vi "pathtracking.vi"(8 "x":dbl, 11 "y":dbl) -> (3 "R":dbl)   [LabVIEW 2012]
uses:
  G_NAV.vi
  G_VEH.vi
  G_PATH.vi
  <vilib>/Analysis/NI_AALBase.lvlib
  <vilib>/Analysis/baseanly.llb/Real Determinant.vi
  <vilib>/Analysis/baseanly.llb/Real Inverse Matrix.vi
  <vilib>/Analysis/baseanly.llb/A x Vector.vi
panel:
  out "Waveform Graph":dbl[](graph)
  out "Array 2":dbl[](array[numeric])
  out "Array":dbl[](array[numeric])
  out "x*y 2":dbl[](array[numeric])
  out "sqrt(x)":dbl[](array[numeric])
  out "x*y":dbl[](array[numeric])
  out "map_track 2":dbl[][](array[numeric])
  out "sum":dbl
  out "M6006":T1={"GPSTime"=22892800.0, "attitude[2]"=-0.6123908, "lcc[0]"=-970.47205, "lcc[1]"=200.52362, "heading_GPS"=-0.6106907} {"GPSTime" format="%#_6f"}
  out "stack":bool=TRUE
  out "lw":dbl=0.4
  out "tic":u32=313769281
  out "reverse":bool
  out "map_track":dbl[][](array[numeric])=[[-0.6687401515638595, -3.551350516814976], [-1.1601880006125764, -3.4580278333550782], [-1.6512488590649952, -3.3629580799680854], [-2.1418835557610314, -3.265964418362822], [-2.6320529195405924, -3.1668700102479344], [-3.12171777924361, -3.0654980173321356], [-3.6108389637099756, -2.961671601324125], [-4.250355012057505, -2.8217269001890974], [-4.733554194697693, -2.693195492254268]]
  out "track":dbl[][](array[numeric])=[[-0.6687401515638595, -3.551350516814976], [-1.1601880006125764, -3.4580278333550782], [-1.6512488590649952, -3.3629580799680854], [-2.1418835557610314, -3.265964418362822], [-2.6320529195405924, -3.1668700102479344], [-3.12171777924361, -3.0654980173321356], [-3.6108389637099756, -2.961671601324125], [-4.250355012057505, -2.8217269001890974], [-4.733554194697693, -2.693195492254268], [-5.215089885143842, -2.558342659026822], [-5.693483406062963, -2.4115492889016945], [-6.167256080122039, -2.24719627027381], [-6.634929229988109, -2.059664491538052], [-7.095024178328142, -1.8433348410893422], [-7.546062247809149, -1.5925882073226139], [-7.98656476109811, -1.301805478632852], [-8.415053040862054, -0.9653675434148765], [-8.830048409767974, -0.5776552900636165], [-9.230072190482858, -0.133049606974057], [-9.61364570567371, 0.3740686174589265], [-9.97929027800753, 0.949318494840405], [-10.386059580111024, 1.7242186788508236], [-10.53357405922493, 2.2019628347040774], [-10.66851200140239, 2.6835902739278463], [-10.772007434080049, 3.1749262819640283], [-10.825194384694537, 3.6817961442544633], [-10.809206880682517, 4.210025146240928], [-10.705178949480636, 4.765438573365376], [-10.494244618525542, 5.353861711069529], [-10.157537915253862, 5.981119844795286], [-9.676192867102248, 6.653038259984428], [-8.946295802610212, 7.461572105302583], [-8.539313408094966, 7.752602995705581], [-8.110420661696207, 8.015244834208291], [-7.660232732059987, 8.25029468946181], [-7.189364787832295, 8.458549630117131], [-6.698431997659123, 8.640806724825243], [-6.188049530186491, 8.797863042237132], [-5.658832554060375, 8.930515651003796], [-5.11139623792681, 9.039561619776274], [-4.546355750431802, 9.12579801720561], [-3.9643262602213256, 9.190021911942688], [-3.3659229359414162, 9.233030372638604], [-2.7517609462380523, 9.25562046794435], [-2.122455459757251, 9.258589266510917], [-1.4786216451450183, 9.242733836989292], [-0.8208746710473604, 9.208851248030518], [-0.1498297061102689, 9.157738568285591], [0.5338980810202378, 9.090192866405497], [1.229693521698167, 9.007011211041284], [1.9369414472775146, 8.908990670843883], [2.6550266891122614, 8.796928314464337], [3.383334078556428, 8.671621210553642], [4.121248446963983, 8.53386642776284], [4.868154625688948, 8.384461034742866], [5.623437446085289, 8.224202100144819], [6.386481739507029, 8.053886692619635], [7.156672337308164, 7.874311880818305], [7.838146127104554, 7.70968069378327], [8.321781606815595, 7.582803343212244], [8.805290536895978, 7.45544776805299], [9.287663918083021, 7.323801011645703], [9.76789275111402, 7.18405011733063], [10.244968036726283, 7.032382128447967], [10.717880775657084, 6.864984088337955], [11.18562196864372, 6.678043040340844], [11.647182616423507, 6.4677460277968315], [12.101553719733744, 6.230280094046104], [12.547726279311707, 5.961832282428966], [12.984691295894704, 5.658589636285609], [13.411439770220039, 5.3167391989562285], [13.939637565704926, 4.818324597988705], [14.177469695018669, 4.377621822306417], [14.370305638929839, 3.9092831916317614], [14.522185803389362, 3.415790251277338], [14.637150594348116, 2.8996245465557346], [14.719240417757044, 2.363267622779441], [14.77249567956704, 1.8092010252611073], [14.800956785728996, 1.2399062993133256], [14.808664142193827, 0.6578649902486369], [14.799658154912459, 0.06555864337958095], [14.777979229835777, -0.5345311959811911]]
  out "xyhc":T2={"c_idx"=71, "xc"=-91.48037348905598, "yc"=-434.27857700428615, "hc"=-0.4484199308552679, "xc_path"=12.43286899562552}
  in  "margin":dbl
  out "vr":dbl=0.75
  out "vf":dbl=3.5
  out "vw":dbl=0.9025
  out "ymax":dbl=12.0
  out "ymin":dbl=-6.0
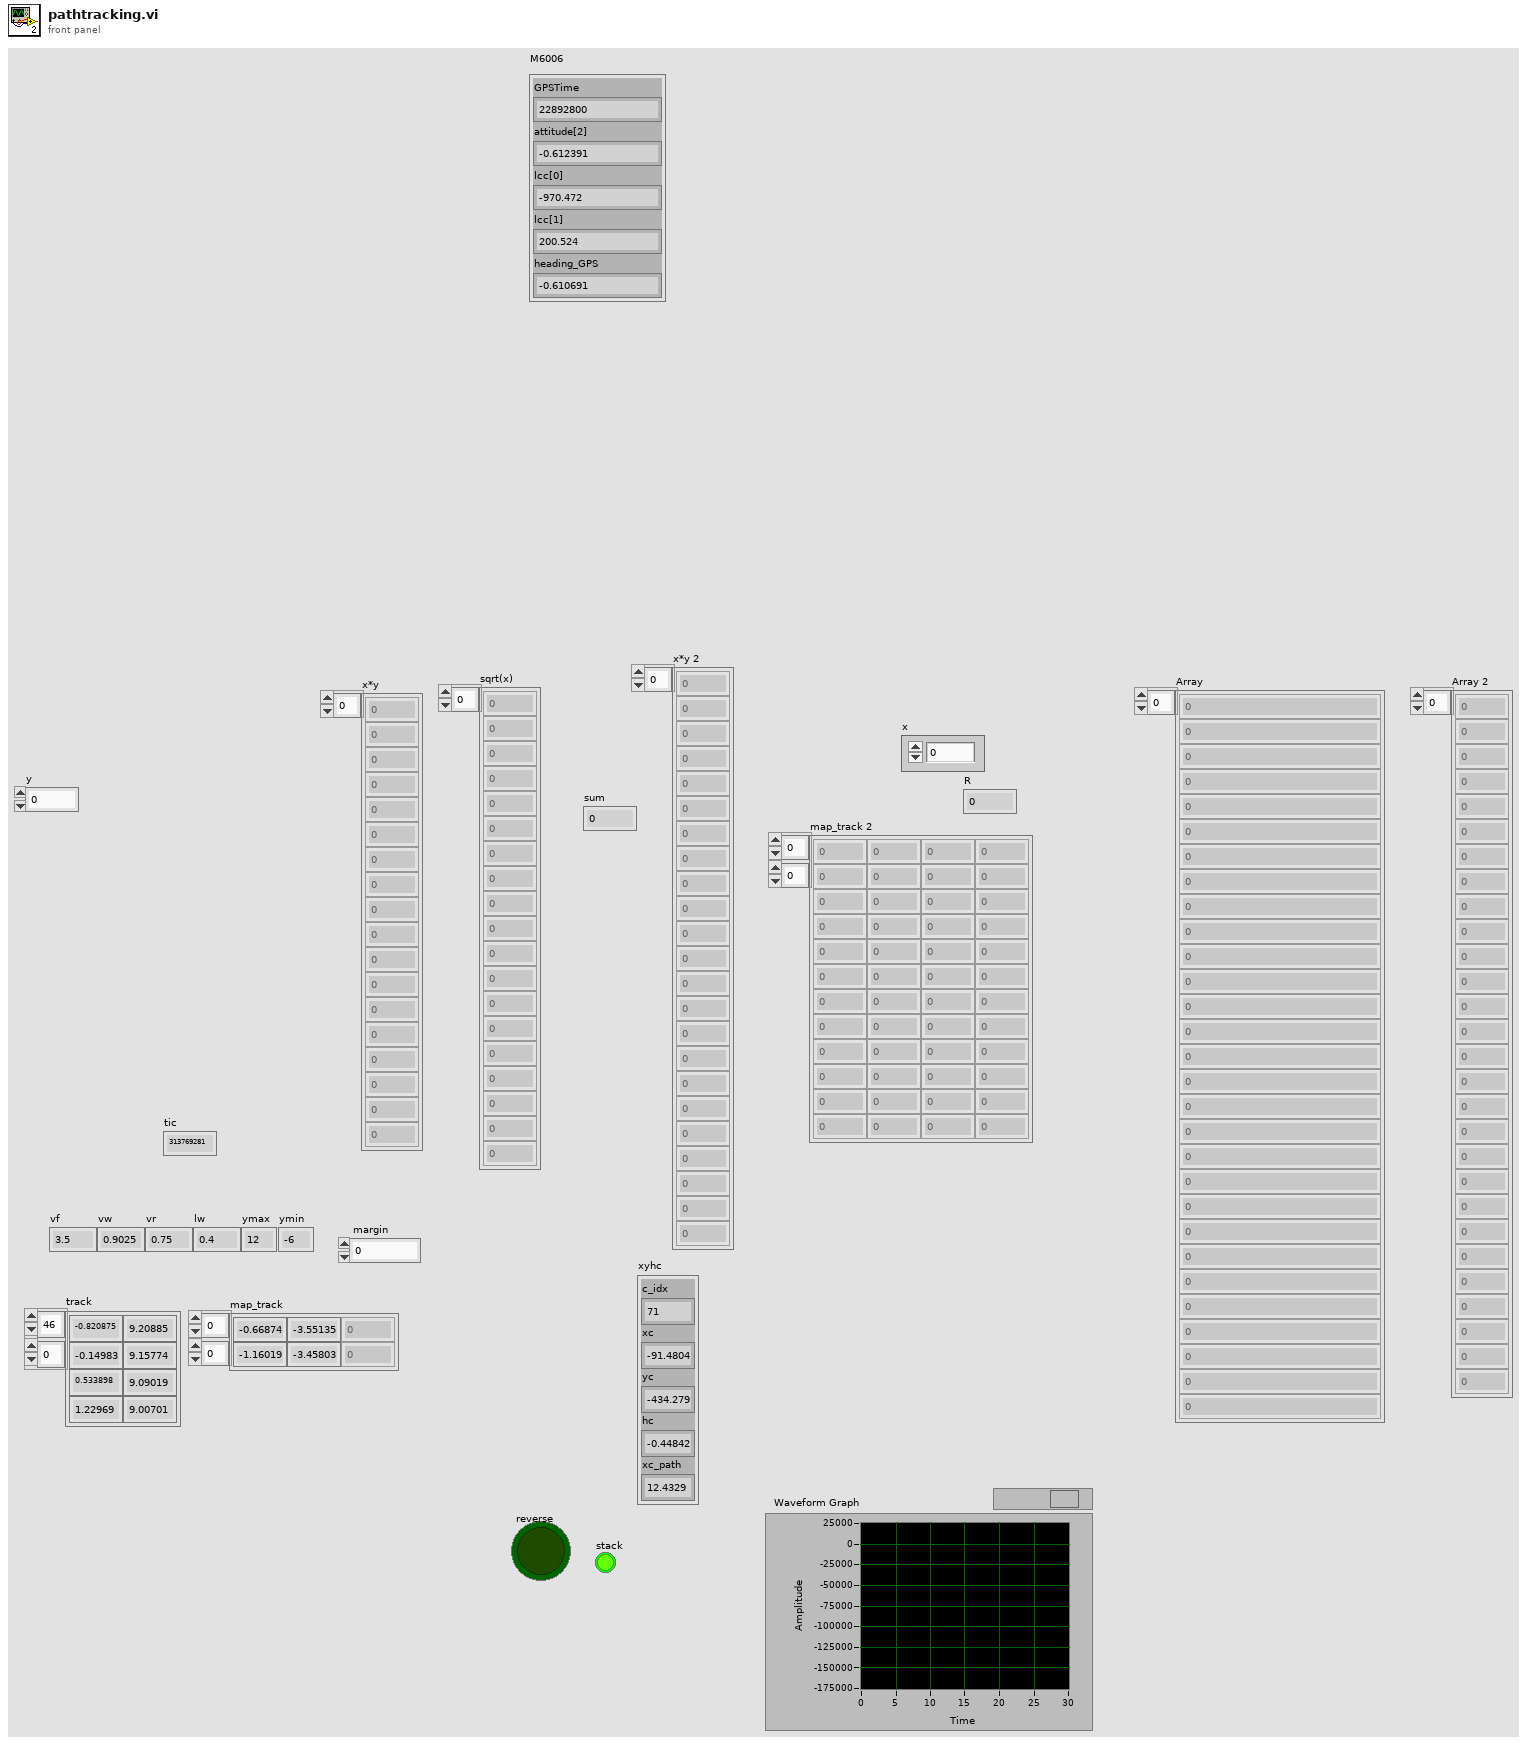
[diagram p1: front panel]
types:
  T1 = cluster{"GPSTime":dbl, "attitude[2]":sgl, "lcc[0]":sgl, "lcc[1]":sgl, "heading_GPS":sgl}
  T2 = cluster{"c_idx":i32, "xc":dbl, "yc":dbl, "hc":dbl, "xc_path":dbl}
  T3 = enum32{"General", "Positive Definite", "Lower Triangular", "Upper Triangular"}
  T4 = cluster{"GPSTime":dbl, "attitude[2]":dbl, "lcc[0]":dbl, "lcc[1]":dbl, "heading_GPS":dbl}
  T5 = cluster{"Steer_input":dbl, "Steer_output":dbl, "VS_des":dbl, "VS_can":dbl, "heading":dbl, "auto":bool, "run":bool, "x":dbl, "y":dbl}
  T6 = cluster{"idx":i32, "x":dbl, "y":dbl, "h":dbl, "x_path":dbl}
  T7 = typedef "NI_Matrix.lvlib/RealMatrix.ctl" = dbl[][]
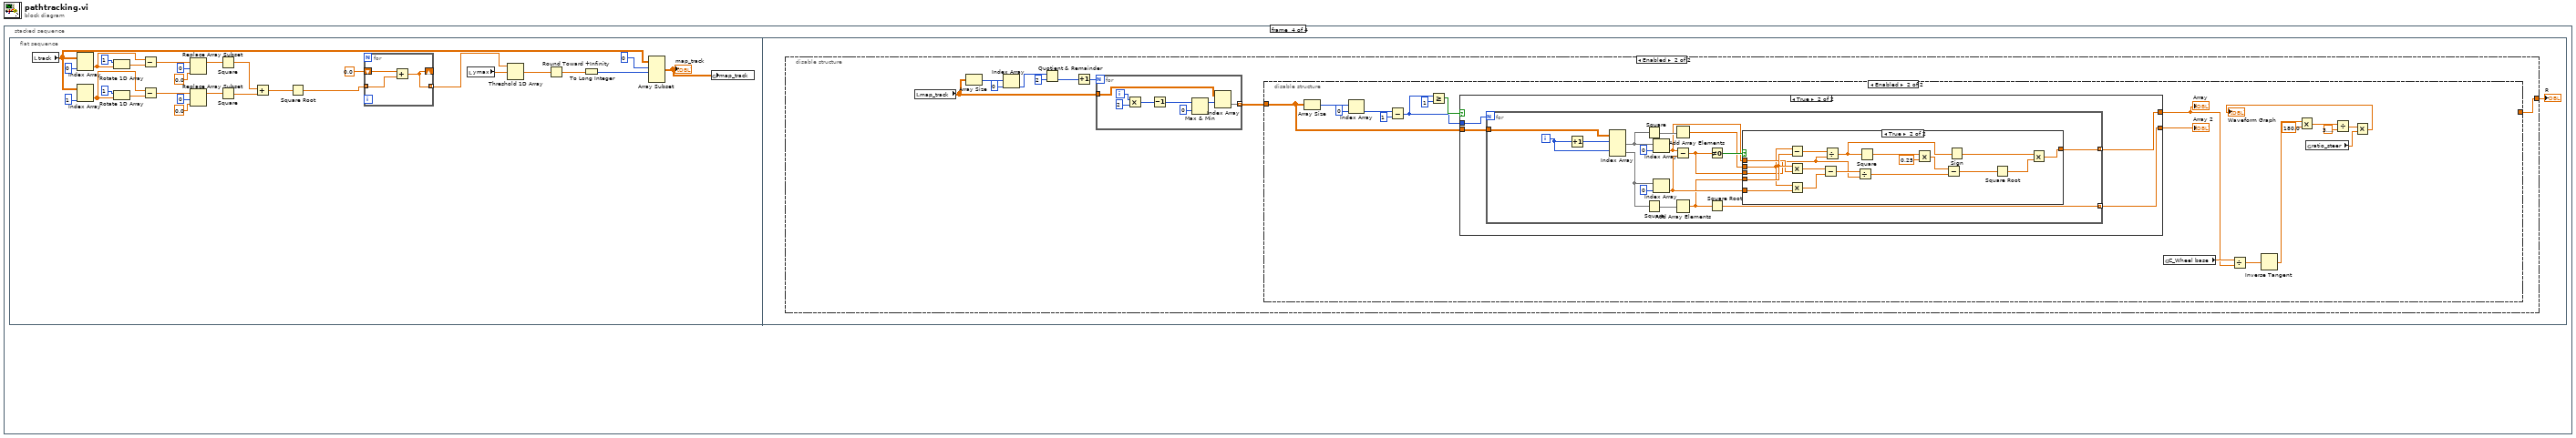
[diagram p0: block diagram]
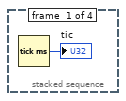
[diagram p2: hidden frame]
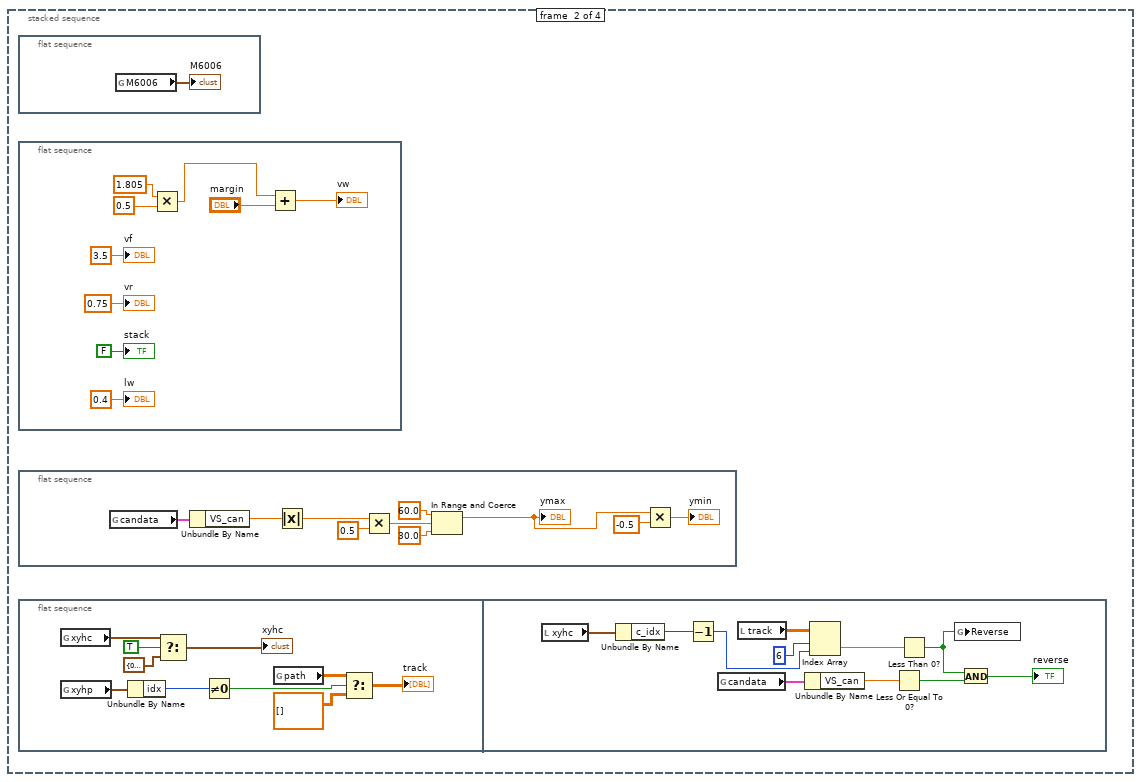
[diagram p3: hidden frame]
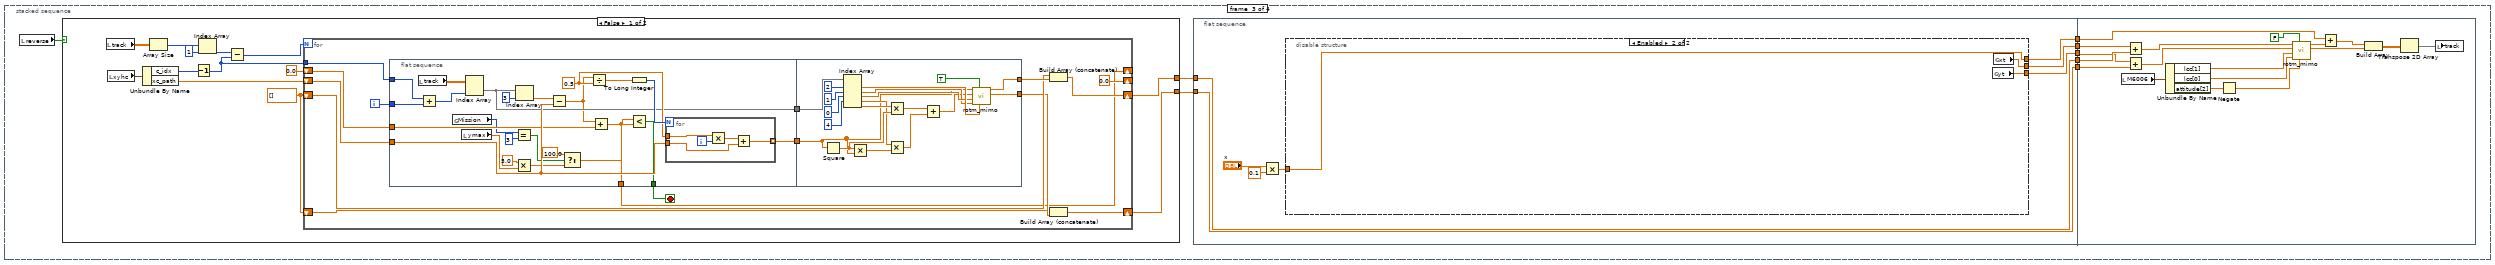
[diagram p4: hidden frame]
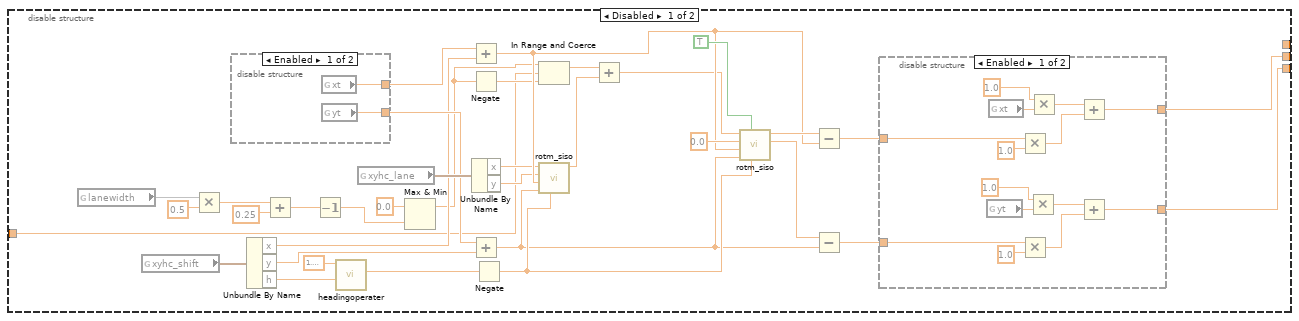
[diagram p5: hidden frame]
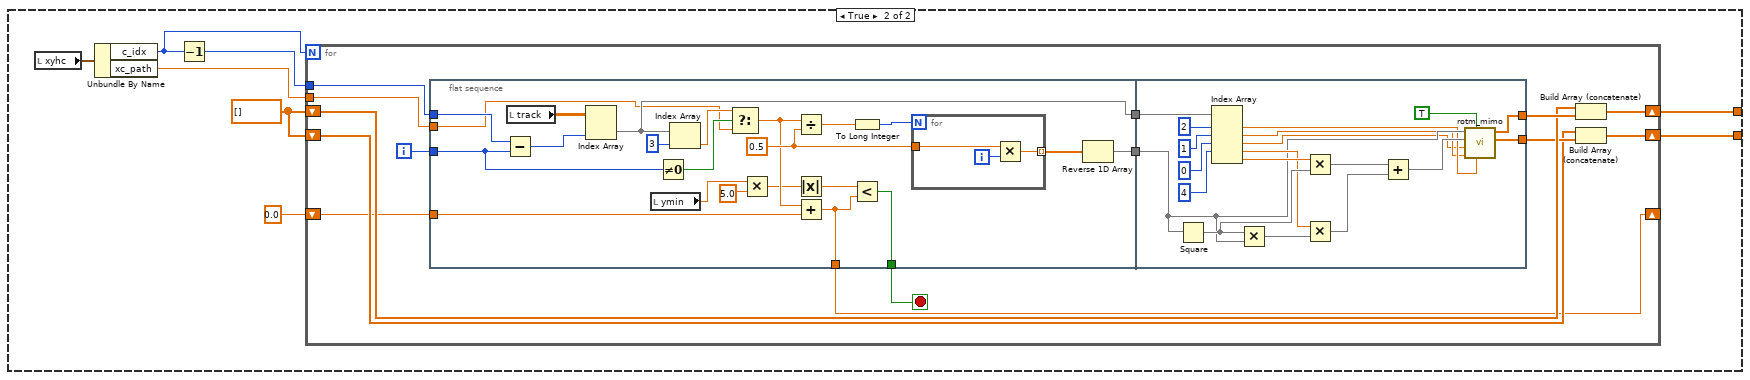
[diagram p8: hidden frame]
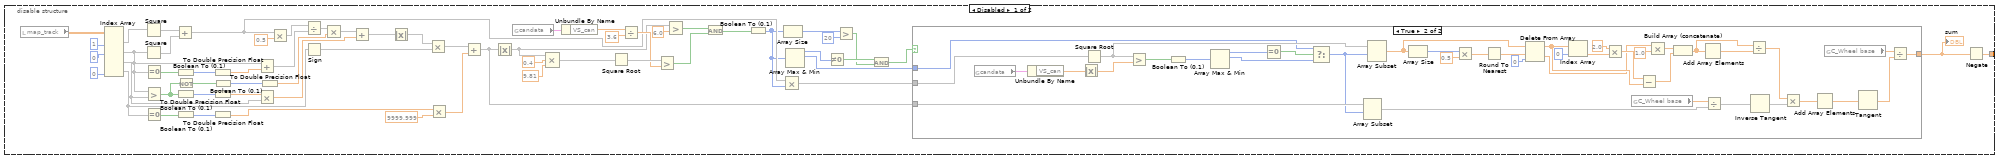
[diagram p9: hidden frame]
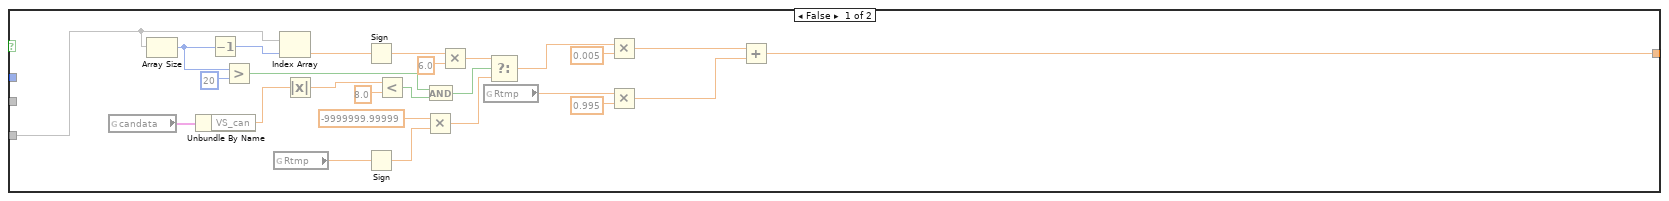
[diagram p10: hidden frame]
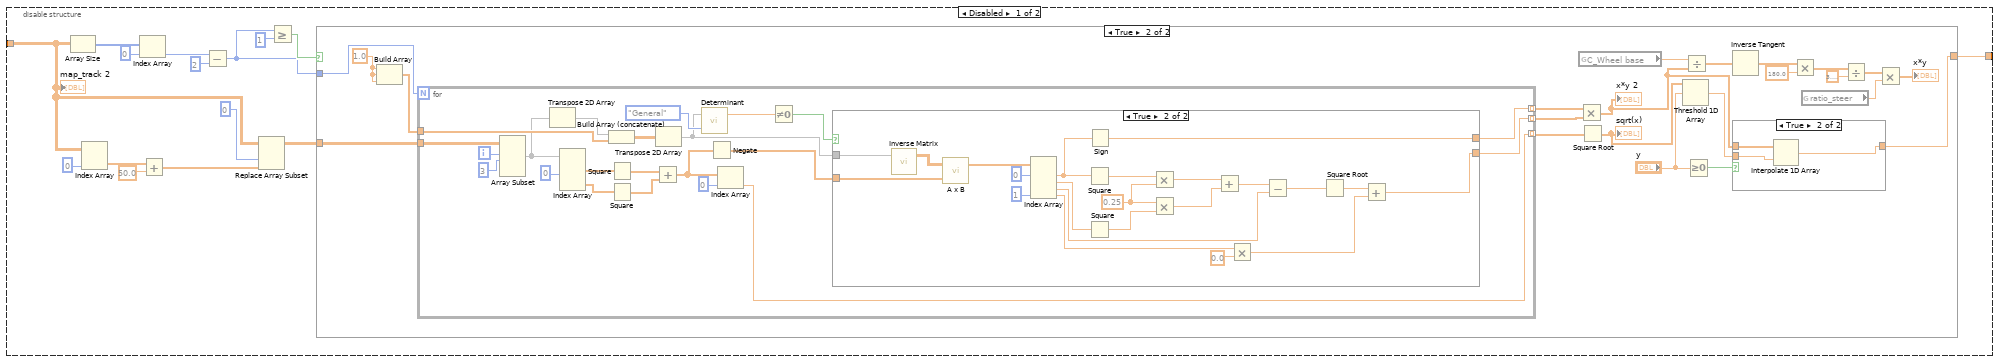
[diagram p11: hidden frame]
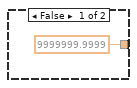
[diagram p12: hidden frame]
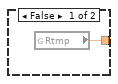
[diagram p13: hidden frame]
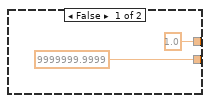
[diagram p14: hidden frame]
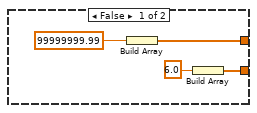
[diagram p15: hidden frame]
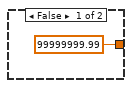
[diagram p16: hidden frame]
diagram:
  n1 = stacked-sequence {
    frame #0 {
      n2 = Tick Count (ms)() -> (millisecond timer value=→"tic":u32)
    }
    frame #1 {
      n3 = flat-sequence {
        frame #0 {
          n4 = global read "G_NAV.vi" "M6006"() -> (→"M6006":T4)
        }
      }
      n5 = flat-sequence {
        frame #0 {
          n6 = Multiply(x=1.805 ("width"), y=0.5) -> (x*y=w24:dbl)
          n7 = Add(x=w24, y="margin") -> (x+y=→"vw":dbl)
          "lw" <- 0.4 ("width")
          "vf" <- 3.5 ("af")
          "vr" <- 0.75 ("ar")
          "stack" <- FALSE
        }
      }
      n8 = flat-sequence {
        frame #0 {
          n9 = global read "G_VEH.vi" "candata"() -> (w41:T5)
          n10 = Unbundle By Name(w41) -> ("VS_can"=w38:dbl)
          n11 = Absolute Value(x=w38) -> (abs(x)=w34:dbl)
          n12 = Multiply(x=w34, y=0.5 ("vgain")) -> (x*y=w33:dbl)
          n13 = In Range and Coerce(upper limit=60.0, x=w33, lower limit=30.0 ("y")) -> (coerced(x)=w37:dbl)  [unwired: 1 out]
          "ymax" <- w37
          n14 = Multiply(x=w37, y=-0.5) -> (x*y=→"ymin":dbl)
        }
      }
      n15 = flat-sequence {
        frame #0 {
          n16 = global read "G_VEH.vi" "xyhc"() -> (w9:T6)
          n17 = global read "G_VEH.vi" "xyhp"() -> (w4:T6)
          n18 = Unbundle By Name(w4) -> ("idx"=w3:i32)
          n19 = Select(t=w9, s=TRUE ("B_track"), f=T2 {"c_idx"=0, "xc"=0.0, "yc"=0.0, "hc"=0.0, "xc_path"=0.0}) -> (s? t:f=→"xyhc":T2)
          n20 = Not Equal To 0?(x=w3) -> (x != 0?=w2:bool)
          n21 = global read "G_PATH.vi" "path"() -> (w5:dbl[][])
          n22 = Select(t=w5, s=w2, f=dbl[][] []) -> (s? t:f=→"track":dbl[][])
        }
        frame #1 {
          n23 = local read "xyhc"() -> (w21:T2)
          n24 = Unbundle By Name(w21) -> ("c_idx"=w19:i32)
          n25 = Decrement(x=w19) -> (x-1=w20:i32)
          n26 = global read "G_VEH.vi" "candata"() -> (w15:T5)
          n27 = local read "track"() -> (w22:dbl[][])
          n28 = Unbundle By Name(w15) -> ("VS_can"=w16:dbl)
          n29 = Index Array(array=w22, index (row)=6, index (col)=w20) -> (element=w17:dbl)
          n30 = Less Or Equal To 0?(x=w16) -> (x <= 0?=w13:bool)
          n31 = Less Than 0?(x=w17) -> (x < 0?=w14:bool)
          n32 = global write "G_VEH.vi" "Reverse"(w14) -> ()
          n33 = And(x=w14, y=w13) -> (x .and. y?=→"reverse":bool)
        }
      }
    }
    frame #2 {
      n34 = local read "reverse"() -> (w48:bool)
      n35 = case shown="False" w48 {
        tunnel: [w136 w211] -> w50
        tunnel: [w135 w210] -> w49
        frame False {
          w138 = dbl[] [] ("x")
          n36 = local read "track"() -> (w133:dbl[][])
          n37 = local read "xyhc"() -> (w132:T2)
          n38 = Unbundle By Name(w132) -> ("c_idx"=w143:i32, "xc_path"=w131:dbl)
          n39 = Array Size(array=w133) -> (size(s)=w142:i32[])
          n40 = Decrement(x=w143) -> (x-1=w139:i32)
          n41 = Index Array(array=w142, index=1) -> (element=w140:i32)
          n42 = Subtract(x=w140, y=w139) -> (x-y=w137:i32)
          n43 = for {
            N: w137 -> [_]
            tunnel: w139 -> [w157]
            shift-right: [0.0 ("xc_path")] -> _
            shift-left: w131 -> [w155]
            shift-right: [w150] -> w136
            shift-left: w138 -> [w151]
            shift-right: [w147] -> w135
            shift-left: w138 -> [w148]
            shift-right: [w145] -> _
            shift-left: 0.0 -> [w146]
            i -> [w158]
            stop <- w144 stop-if-true
            n44 = flat-sequence {
              tunnel: w158 -> [w182]
              tunnel: w157 -> [w181]
              tunnel: w155 -> [w175]
              tunnel: [w173] -> w154
              tunnel: [w172] -> w153
              tunnel: w146 -> [w170]
              tunnel: [w169] -> w145
              tunnel: [w168] -> w144
              tunnel: w154 -> [w188]
              tunnel: w153 -> [w199]
              tunnel: [w195] -> w152
              tunnel: [w194] -> w149
              frame #0 {
                w174 = 0.5 ("y")
                n45 = local read "track"() -> (w167:dbl[][])
                n46 = Add(x=w181, y=w182) -> (x+y=w180:i32)
                n47 = global read "G_PATH.vi" "Mission"() -> (w159:i32)
                n48 = local read "ymax"() -> (w166:dbl)
                n49 = Index Array(array=w167, index (col)=w180) -> (element=w172:dbl[])  [unwired: 1 in]
                n50 = Equal?(x=w159, y=3) -> (x = y?=w164:bool)
                n51 = Multiply(x=5.0 ("f"), y=w166) -> (x*y=w161:dbl)
                n52 = Index Array(array=w172, index=3) -> (element=w178:dbl)
                n53 = Subtract(x=w178, y=w175) -> (x-y=w171:dbl)
                n54 = Select(t=100.0 ("x"), s=w164, f=w161) -> (s? t:f=w160:dbl)
                n55 = Divide(x=w171, y=w174) -> (x/y=w177:dbl)
                n56 = Add(x=w171, y=w170) -> (x+y=w169:dbl)
                n57 = To Long Integer(number=w177) -> (32bit integer=w176:i32)
                n58 = Less?(x=w160, y=w169) -> (x < y?=w168:bool)
                n59 = for {
                  N: w176 -> [_]
                  tunnel: w175 -> [w183]
                  tunnel: w174 -> [w186]
                  tunnel: [w185] -> w173 mode=indexing
                  i -> [w187]
                  n60 = Multiply(x=w186, y=w187) -> (x*y=w184:dbl)
                  n61 = Add(x=w184, y=w183) -> (x+y=w185:dbl)
                }
              }
              frame #1 {
                n62 = Square(x=w188) -> (x^2=w204:dbl[])
                n63 = Index Array(array=w199, index #1=2 ("index"), index #2=1 ("index"), index #3=0 ("index"), index #4=4 ("index")) -> (element #1=w192:dbl, element #2=w190:dbl, element #3=w191:dbl, element #4=w203:dbl, element #5=w205:dbl)  [unwired: 1 in]
                n64 = Multiply(x=w204, y=w188) -> (x*y=w202:dbl[])
                n65 = Multiply(x=w205, y=w204) -> (x*y=w201:dbl[])
                n66 = Multiply(x=w203, y=w202) -> (x*y=w200:dbl[])
                n67 = Add(x=w201, y=w200) -> (x+y=w189:dbl[])
                n68 = call "rotm_mimo.vi"("angle[rad]"=w192, "reverse"=TRUE, "y0"=w190, "x0"=w191, "y"=w189, "x"=w188) -> ("Y"=w194:dbl[], "X"=w195:dbl[])  [unwired: 2 in, 2 out]
              }
            }
            n69 = Build Array (concatenate)(w151, w152) -> (w150:dbl[])
            n70 = Build Array (concatenate)(w148, w149) -> (w147:dbl[])
          }
        }
        frame True {
          w212 = dbl[] [] ("x")
          n71 = local read "xyhc"() -> (w207:T2)
          n72 = Unbundle By Name(w207) -> ("c_idx"=w209:i32, "xc_path"=w213:dbl)
          n73 = Decrement(x=w209) -> (x-1=w214:i32)
          n74 = for {
            N: w209 -> [_]
            tunnel: w214 -> [w227]
            shift-right: [w221] -> w211
            shift-left: w212 -> [w222]
            shift-right: [w218] -> w210
            shift-left: w212 -> [w219]
            tunnel: w213 -> [w226]
            shift-right: [w216] -> _
            shift-left: 0.0 -> [w217]
            i -> [w228]
            stop <- w215 stop-if-true
            n75 = flat-sequence {
              tunnel: w228 -> [w243]
              tunnel: w227 -> [w250]
              tunnel: w226 -> [w240]
              tunnel: [w238] -> w225
              tunnel: [w244] -> w224
              tunnel: w217 -> [w236]
              tunnel: [w235] -> w216
              tunnel: [w234] -> w215
              tunnel: w225 -> [w258]
              tunnel: w224 -> [w265]
              tunnel: [w261] -> w223
              tunnel: [w260] -> w220
              frame #0 {
                w245 = 0.5 ("y")
                n76 = Subtract(x=w250, y=w243) -> (x-y=w249:i32)
                n77 = local read "track"() -> (w233:dbl[][])
                n78 = Index Array(array=w233, index (col)=w249) -> (element=w244:dbl[])  [unwired: 1 in]
                n79 = local read "ymin"() -> (w231:dbl)
                n80 = Not Equal To 0?(x=w243) -> (x != 0?=w242:bool)
                n81 = Index Array(array=w244, index=3) -> (element=w241:dbl)
                n82 = Select(t=w241, s=w242, f=w240) -> (s? t:f=w237:dbl)
                n83 = Multiply(x=w231, y=5.0) -> (x*y=w230:dbl)
                n84 = Divide(x=w237, y=w245) -> (x/y=w247:dbl)
                n85 = Absolute Value(x=w230) -> (abs(x)=w232:dbl)
                n86 = Add(x=w237, y=w236) -> (x+y=w235:dbl)
                n87 = To Long Integer(number=w247) -> (32bit integer=w246:i32)
                n88 = Less?(x=w232, y=w235) -> (x < y?=w234:bool)
                n89 = for {
                  N: w246 -> [_]
                  tunnel: w245 -> [w252]
                  tunnel: [w251] -> w239 mode=indexing
                  i -> [w253]
                  n90 = Multiply(x=w252, y=w253) -> (x*y=w251:dbl)
                }
                n91 = Reverse 1D Array(array=w239) -> (reversed array=w238:dbl[])
              }
              frame #1 {
                n92 = Square(x=w258) -> (x^2=w270:dbl[])
                n93 = Index Array(array=w265, index #1=2 ("index"), index #2=1 ("index"), index #3=0 ("index"), index #4=4 ("index")) -> (element #1=w256:dbl, element #2=w255:dbl, element #3=w254:dbl, element #4=w269:dbl, element #5=w271:dbl)  [unwired: 1 in]
                n94 = Multiply(x=w270, y=w258) -> (x*y=w268:dbl[])
                n95 = Multiply(x=w271, y=w270) -> (x*y=w267:dbl[])
                n96 = Multiply(x=w269, y=w268) -> (x*y=w266:dbl[])
                n97 = Add(x=w267, y=w266) -> (x+y=w259:dbl[])
                n98 = call "rotm_mimo.vi"("angle[rad]"=w256, "reverse"=TRUE, "y0"=w255, "x0"=w254, "y"=w259, "x"=w258) -> ("Y"=w260:dbl[], "X"=w261:dbl[])  [unwired: 2 in, 2 out]
              }
            }
            n99 = Build Array (concatenate)(w222, w223) -> (w221:dbl[])
            n100 = Build Array (concatenate)(w219, w220) -> (w218:dbl[])
          }
        }
      }
      n101 = flat-sequence {
        tunnel: w49 -> [w57]
        tunnel: w50 -> [w58]
        tunnel: [w58] -> w47
        tunnel: [w57] -> w46
        tunnel: [w56] -> w45
        tunnel: [w55] -> w44
        tunnel: [w51] -> w43
        tunnel: w47 -> [w121]
        tunnel: w46 -> [w119]
        tunnel: w45 -> [w117]
        tunnel: w44 -> [w116]
        tunnel: w43 -> [w114]
        frame #0 {
          n102 = Multiply(x="x", y=0.1) -> (x*y=w52:dbl)
          n103 = disable-structure shown="Enabled" {
            disable-tunnel: [w66 w112] -> w56
            disable-tunnel: [w65 w111] -> w55
            disable-tunnel: w52 -> [w61 w110]
            disable-tunnel: [_ w110] -> w51
            frame Disabled {
              n104 = global read "G_PATH.vi" "lanewidth"() -> (w59)
              n105 = global read "G_VEH.vi" "xyhc_shift"() -> (w74:T6)
              n106 = Multiply(x=w59, y=0.5) -> (x*y=w64:dbl)
              n107 = disable-structure shown="Enabled" {
                disable-tunnel: [w109 _] -> w78
                disable-tunnel: [w108 _] -> w80
                frame Enabled {
                  n108 = global read "G_PATH.vi" "xt"() -> (w109:dbl)
                  n109 = global read "G_PATH.vi" "yt"() -> (w108:dbl)
                }
                frame Disabled {
                }
              }
              n110 = Unbundle By Name(w74) -> ("x"=w77:dbl, "y"=w79:dbl, "h"=w83:dbl)
              n111 = Add(x=w64, y=0.25) -> (x+y=w62:dbl)
              n112 = Decrement(x=w62) -> (x-1=w69:dbl)
              n113 = call "headingoperater.vi"("h1"=w83, "h2"=1.5707963267948966) -> ("h2-h1"=w91:dbl)  [unwired: 8 in, 1 out]
              n114 = global read "G_VEH.vi" "xyhc_lane"() -> (w93:T6)
              n115 = Max & Min(x=0.0, y=w69) -> (max(x,y)=w68:dbl)  [unwired: 1 out]
              n116 = Add(x=w78, y=w77) -> (x+y=w85:dbl)
              n117 = Negate(x=w68) -> (-x=w67:dbl)
              n118 = Add(x=w80, y=w79) -> (x+y=w86:dbl)
              n119 = Unbundle By Name(w93) -> ("x"=w76:dbl, "y"=w75:dbl)
              n120 = Negate(x=w91) -> (-x=w92:dbl)
              n121 = In Range and Coerce(upper limit=w68, x=w61, lower limit=w67) -> (coerced(x)=w60:dbl)  [unwired: 1 out]
              n122 = call "rotm_siso.vi"("angle[rad]"=w92, "y0"=w86, "x0"=w85, "y"=w75, "x"=w76) -> ("x'"=w73:dbl)  [unwired: 5 in, 1 out]
              n123 = Add(x=w60, y=w73) -> (x+y=w72:dbl)
              n124 = call "rotm_siso.vi"("angle[rad]"=w92, "reverse"=TRUE, "y0"=w86, "x0"=w85, "y"=0.0, "x"=w72) -> ("y'"=w89:dbl, "x'"=w88:dbl)  [unwired: 4 in]
              n125 = Subtract(x=w88, y=w85) -> (x-y=w81:dbl)
              n126 = Subtract(x=w89, y=w86) -> (x-y=w82:dbl)
              n127 = disable-structure shown="Enabled" {
                disable-tunnel: w81 -> [w103 _]
                disable-tunnel: w82 -> [w97 _]
                disable-tunnel: [w95 _] -> w66
                disable-tunnel: [w94 _] -> w65
                frame Enabled {
                  n128 = global read "G_PATH.vi" "yt"() -> (w100:dbl)
                  n129 = global read "G_PATH.vi" "xt"() -> (w107:dbl)
                  n130 = Multiply(x=w103, y=1.0 ("x")) -> (x*y=w102:dbl)
                  n131 = Multiply(x=w97, y=1.0 ("x")) -> (x*y=w96:dbl)
                  n132 = Multiply(x=1.0, y=w100) -> (x*y=w99:dbl)
                  n133 = Multiply(x=1.0, y=w107) -> (x*y=w105:dbl)
                  n134 = Add(x=w105, y=w102) -> (x+y=w95:dbl)
                  n135 = Add(x=w99, y=w96) -> (x+y=w94:dbl)
                }
                frame Disabled {
                }
              }
            }
            frame Enabled {
              n136 = global read "G_PATH.vi" "yt"() -> (w111:dbl)
              n137 = global read "G_PATH.vi" "xt"() -> (w112:dbl)
            }
          }
        }
        frame #1 {
          n138 = local read "M6006"() -> (w123:T1)
          n139 = Add(x=w117, y=w121) -> (x+y=w120:dbl[])
          n140 = Add(x=w116, y=w119) -> (x+y=w118:dbl[])
          n141 = Unbundle By Name(w123) -> ("lcc[1]"=w127:sgl, "lcc[0]"=w126:sgl, "attitude[2]"=w122:sgl)
          n142 = Negate(x=w122) -> (-x=w124:sgl)
          n143 = call "rotm_mimo.vi"("angle[rad]"=w124, "reverse"=FALSE, "y0"=w126, "x0"=w127, "y"=w118, "x"=w120) -> ("Y"=w129:dbl[], "X"=w115:dbl[])  [unwired: 2 in, 2 out]
          n144 = Add(x=w114, y=w115) -> (x+y=w113:dbl[])
          n145 = Build Array(w113, w129) -> (w128:dbl[][])
          n146 = Transpose 2D Array(2D array=w128) -> (transposed array=w130:dbl[][])
          n147 = local write "track"(w130) -> ()
        }
      }
    }
    frame #3 {
      n148 = flat-sequence {
        frame #0 {
          n149 = local read "track"() -> (w274:dbl[][])
          n150 = Index Array(array=w274, index (col)=0 ("disabled index (col)")) -> (element=w298:dbl[])  [unwired: 1 in]
          n151 = Index Array(array=w274, index (col)=1 ("disabled index (col)")) -> (element=w287:dbl[])  [unwired: 1 in]
          n152 = Rotate 1D Array(1:w298, 2:1 ("n")) -> (0:w297:dbl[])
          n153 = Rotate 1D Array(1:w287, 2:1 ("n")) -> (0:w288:dbl[])
          n154 = Subtract(x=w298, y=w297) -> (x-y=w296:dbl[])
          n155 = Subtract(x=w287, y=w288) -> (x-y=w289:dbl[])
          n156 = Replace Array Subset(array=w296, new element=0.0 ("new element/subarray"), index=0) -> (w293:dbl[])
          n157 = Replace Array Subset(array=w289, new element=0.0 ("new element/subarray"), index=0) -> (w292:dbl[])
          n158 = Square(x=w293) -> (x^2=w284:dbl[])
          n159 = Square(x=w292) -> (x^2=w283:dbl[])
          n160 = Add(x=w284, y=w283) -> (x+y=w282:dbl[])
          n161 = Square Root(x=w282) -> (sqrt(x)=w281:dbl[])
          n162 = for {
            tunnel: w281 -> [w304] mode=indexing
            shift-right: [w302] -> _
            shift-left: 0.0 -> [w303]
            tunnel: [w302] -> w275 mode=indexing
            n163 = Add(x=w303, y=w304) -> (x+y=w302:dbl)
          }
          n164 = local read "ymax"() -> (w279:dbl)
          n165 = Threshold 1D Array(2:w279, 3:w275) -> (0:w278:dbl)  [unwired: 1 in]
          n166 = Round Toward +Infinity(x=w278) -> (ceil(x): smallest int >= x=w277:dbl)
          n167 = To Long Integer(number=w277) -> (32bit integer=w301:i32)
          n168 = Array Subset(array=w274, index (row)=0 ("index"), length (row)=w301) -> (w273:dbl[][])  [unwired: 2 in]
          "map_track" <- w273
          n169 = global write "G_PATH.vi" "map_track"(w273) -> ()
        }
        frame #1 {
          n170 = disable-structure shown="Enabled" {
            disable-tunnel: [w306 w433] -> w305
            frame Disabled {
              n171 = local read "map_track"() -> (w365:dbl[][])
              n172 = Index Array(array=w365, index (col) #1=1 ("disabled index (col)"), index (col) #2=0 ("disabled index (col)"), index (col) #4=0 ("index (col)")) -> (element #1=w355:dbl[], element #2=w342:dbl[], element #3=w361:dbl[], element #4=w336:dbl[])  [unwired: 5 in]
              n173 = Square(x=w355) -> (x^2=w354:dbl[])
              n174 = Square(x=w342) -> (x^2=w353:dbl[])
              n175 = Equal To 0?(x=w342) -> (x = 0?=w344:bool[])
              n176 = Greater?(x=w342, y=w361) -> (0:w359:bool[])
              n177 = Equal To 0?(x=w336) -> (x = 0?=w338:bool[])
              n178 = Add(x=w354, y=w353) -> (x+y=w318:dbl[])
              n179 = Boolean To (0,1)(Boolean=w344) -> (0, 1=w345:i16[])
              n180 = Not(x=w359) -> (.not. x?=w357:bool[])
              n181 = Boolean To (0,1)(Boolean=w359) -> (0, 1=w363:i16[])
              n182 = Boolean To (0,1)(Boolean=w338) -> (0, 1=w337:i16[])
              n183 = To Double Precision Float(number=w345) -> (double precision float=w343:dbl[])
              n184 = Boolean To (0,1)(Boolean=w357) -> (0, 1=w358:i16[])
              n185 = To Double Precision Float(number=w363) -> (double precision float=w362:dbl[])
              n186 = To Double Precision Float(number=w337) -> (double precision float=w335:dbl[])
              n187 = Add(x=w342, y=w343) -> (x+y=w341:dbl[])
              n188 = Multiply(x=w362, y=w361) -> (x*y=w360:dbl[])
              n189 = To Double Precision Float(number=w358) -> (double precision float=w349:dbl[])
              n190 = Multiply(x=w318, y=0.5) -> (x*y=w351:dbl[])
              n191 = Divide(x=w351, y=w341) -> (x/y=w350:dbl[])
              n192 = Sign(1:w336) -> (0:w339:dbl[])
              n193 = Multiply(x=w350, y=w349) -> (x*y=w348:dbl[])
              n194 = Add(x=w348, y=w360) -> (x+y=w347:dbl[])
              n195 = Absolute Value(x=w347) -> (abs(x)=w340:dbl[])
              n196 = Multiply(x=w340, y=w339) -> (x*y=w333:dbl[])
              n197 = Multiply(x=w335, y=9999.999) -> (x*y=w332:dbl[])
              n198 = Add(x=w333, y=w332) -> (x+y=w320:dbl[])
              n199 = Absolute Value(x=w320) -> (abs(x)=w325:dbl[])
              n200 = global read "G_VEH.vi" "candata"() -> (w315:T5)
              n201 = Compound Arithmetic op=MULTIPLY(w325, 0.4 ("value"), 9.81 ("y")) -> (w329:dbl[])
              n202 = Unbundle By Name(w315) -> ("VS_can"=w314:dbl)
              n203 = Square Root(x=w329) -> (sqrt(x)=w328:dbl[])
              n204 = Divide(x=w314, y=3.6) -> (x/y=w327:dbl)
              n205 = Greater?(x=w328, y=w327) -> (0:w322:bool[])
              n206 = Greater?(x=w325, y=6.0) -> (0:w323:bool[])
              n207 = And(x=w323, y=w322) -> (x .and. y?=w321:bool[])
              n208 = Boolean To (0,1)(Boolean=w321) -> (0, 1=w312:i16[])
              n209 = Multiply(x=w318, y=w312) -> (x*y=w317:dbl[])
              n210 = Array Size(array=w312) -> (size(s)=w311:i32)
              n211 = Array Max & Min(array=w312) -> (max value=w326:i16, max index (indices)=w319:i32)  [unwired: 2 out]
              n212 = Not Equal To 0?(x=w326) -> (x != 0?=w309:bool)
              n213 = Greater?(x=w311, y=20) -> (0:w307:bool)
              n214 = And(x=w309, y=w307) -> (x .and. y?=w308:bool)
              n215 = case shown="True" w308 {
                tunnel: w320 -> [w390 w431]
                tunnel: w319 -> [_ w393]
                tunnel: w317 -> [_ w430]
                tunnel: [w383 w407] -> w316
                frame False {
                  n216 = global read "G_VEH.vi" "candata"() -> (w379:T5)
                  n217 = Array Size(array=w390) -> (size(s)=w381:i32)
                  n218 = Unbundle By Name(w379) -> ("VS_can"=w378:dbl)
                  n219 = Decrement(x=w381) -> (x-1=w391:i32)
                  n220 = Greater?(x=w381, y=20) -> (0:w374:bool)
                  n221 = global read "G_VEH.vi" "Rtmp"() -> (w369:dbl)
                  n222 = Index Array(array=w390, index=w391) -> (element=w389:dbl)
                  n223 = Absolute Value(x=w378) -> (abs(x)=w377:dbl)
                  n224 = Sign(1:w389) -> (0:w380:dbl)
                  n225 = Sign(1:w369) -> (0:w367:dbl)
                  n226 = Less?(x=w377, y=8.0) -> (x < y?=w375:bool)
                  n227 = Multiply(x=-9999999.99999, y=w367) -> (x*y=w366:dbl)
                  n228 = And(x=w374, y=w375) -> (x .and. y?=w373:bool)
                  n229 = Multiply(x=w380, y=6.0) -> (x*y=w371:dbl)
                  n230 = global read "G_VEH.vi" "Rtmp"() -> (w388:dbl)
                  n231 = Select(t=w371, s=w373, f=w366) -> (s? t:f=w370:dbl)
                  n232 = Multiply(x=w370, y=0.005) -> (x*y=w385:dbl)
                  n233 = Multiply(x=w388, y=0.995) -> (x*y=w384:dbl)
                  n234 = Add(x=w385, y=w384) -> (x+y=w383:dbl)
                }
                frame True {
                  n235 = global read "G_VEH.vi" "candata"() -> (w402:T5)
                  n236 = Unbundle By Name(w402) -> ("VS_can"=w400:dbl)
                  n237 = Absolute Value(x=w400) -> (abs(x)=w399:dbl)
                  n238 = Square Root(x=w430) -> (sqrt(x)=w401:dbl[])
                  n239 = Greater?(x=w401, y=w399) -> (0:w398:bool[])
                  n240 = Boolean To (0,1)(Boolean=w398) -> (0, 1=w397:i16[])
                  n241 = Array Max & Min(array=w397) -> (max value=w396:i16, max index (indices)=w394:i32)  [unwired: 2 out]
                  n242 = Equal To 0?(x=w396) -> (x = 0?=w395:bool)
                  n243 = Select(t=w393, s=w395, f=w394) -> (s? t:f=w392:i32)
                  n244 = Array Subset(array=w431, index=w392) -> (w414:dbl[])  [unwired: 1 in]
                  n245 = Array Subset(array=w401, index=w392) -> (w425:dbl[])  [unwired: 1 in]
                  n246 = Array Size(array=w425) -> (size(s)=w428:i32)
                  n247 = Multiply(x=w428, y=0.5) -> (x*y=w427:dbl)
                  n248 = Round To Nearest(number=w427) -> (nearest integer value=w426:dbl)
                  n249 = Delete From Array(array=w425, length=w426, index=0) -> (deleted portion=w406:dbl[], array with subset deleted=w419:dbl[])
                  n250 = Index Array(array=w419, index=0) -> (element=w422:dbl)
                  n251 = Multiply(x=2.0, y=w422) -> (x*y=w420:dbl)
                  n252 = global read "G_VEH.vi" "C_Wheel base"() -> (w415:dbl)
                  n253 = Subtract(x=w420, y=w419) -> (x-y=w418:dbl[])
                  n254 = Multiply(x=w406, y=1.0) -> (x*y=w405:dbl[])
                  n255 = Build Array (concatenate)(w405, w418) -> (w416:dbl[])
                  n256 = Add Array Elements(numeric array=w416) -> (sum=w417:dbl)
                  n257 = Divide(x=w415, y=w414) -> (x/y=w413:dbl[])
                  n258 = Divide(x=w416, y=w417) -> (x/y=w403:dbl[])
                  n259 = Inverse Tangent(1:w413) -> (0:w410:dbl[])
                  n260 = Multiply(x=w403, y=w410) -> (x*y=w409:dbl[])
                  n261 = Add Array Elements(numeric array=w409) -> (sum=w408:dbl)
                  n262 = global read "G_VEH.vi" "C_Wheel base"() -> (w411:dbl)
                  n263 = Tangent(1:w408) -> (0:w412:dbl)
                  n264 = Divide(x=w411, y=w412) -> (x/y=w407:dbl)
                }
              }
              "sum" <- w316
              n265 = Negate(x=w316) -> (-x=w306:dbl)
            }
            frame Enabled {
              n266 = local read "map_track"() -> (w436:dbl[][])
              n267 = Array Size(array=w436) -> (size(s)=w440:i32[])
              n268 = Index Array(array=w440, index=0) -> (element=w438:i32)
              n269 = Quotient & Remainder(x=w438, y=2) -> (floor(x/y)=w435:i32)  [unwired: 1 out]
              n270 = Increment(x=w435) -> (x+1=w434:i32)
              n271 = for {
                N: w434 -> [_]
                tunnel: w436 -> [w598]
                tunnel: [w597] -> w432 mode=indexing
                i -> [w592]
                n272 = Multiply(x=w592, y=2) -> (x*y=w596:i32)
                n273 = Decrement(x=w596) -> (x-1=w595:i32)
                n274 = Max & Min(x=w595, y=0) -> (max(x,y)=w594:i32)  [unwired: 1 out]
                n275 = Index Array(array=w598, index (row)=w594) -> (element=w597:dbl[])  [unwired: 1 in]
              }
              n276 = disable-structure shown="Enabled" {
                disable-tunnel: [w448 _] -> w433
                disable-tunnel: w432 -> [w444 w540]
                frame Disabled {
                  n277 = Array Size(array=w444) -> (size(s)=w455:i32[])
                  n278 = Index Array(array=w444, index (col)=0 ("disabled index (col)")) -> (element=w446:dbl[])  [unwired: 1 in]
                  n279 = Index Array(array=w455, index=0) -> (element=w453:i32)
                  n280 = Add(x=w446, y=50.0) -> (x+y=w442:dbl[])
                  n281 = Subtract(x=w453, y=2) -> (x-y=w449:i32)
                  n282 = Replace Array Subset(array=w444, new element=w442, index (col)=0 ("disabled index (col)")) -> (w443:dbl[][])  [unwired: 1 in]
                  n283 = Greater Or Equal?(x=w449, y=1) -> (x >= y?=w450:bool)
                  n284 = case shown="True" w450 {
                    tunnel: w443 -> [_ w478]
                    tunnel: w449 -> [_ w457]
                    tunnel: [9999999.9999 w473] -> w448
                    frame False {
                    }
                    frame True {
                      w477 = 1.0 ("element")
                      n285 = Build Array(w477, w477, w477) -> (w476:dbl[])
                      n286 = for {
                        N: w457 -> [_]
                        tunnel: w478 -> [w504]
                        tunnel: w476 -> [w501]
                        tunnel: [w487] -> w474 mode=indexing
                        tunnel: [w486] -> w475 mode=indexing
                        tunnel: [w483] -> w470 mode=indexing
                        i -> [w503]
                        n287 = Array Subset(array=w504, index (row)=w503, length (row)=3 ("length")) -> (w495:dbl[][])  [unwired: 2 in]
                        n288 = Transpose 2D Array(2D array=w495) -> (transposed array=w500:dbl[][])
                        n289 = Index Array(array=w495, index (col) #1=0 ("disabled index (col)")) -> (element #1=w493:dbl[], element #2=w492:dbl[])  [unwired: 3 in]
                        n290 = Build Array (concatenate)(w500, w501) -> (w499:dbl[][])
                        n291 = Square(x=w493) -> (x^2=w491:dbl[])
                        n292 = Square(x=w492) -> (x^2=w490:dbl[])
                        n293 = Add(x=w491, y=w490) -> (x+y=w485:dbl[])
                        n294 = Transpose 2D Array(2D array=w499) -> (transposed array=w489:dbl[][])
                        n295 = call-poly <vilib>:"Determinant.vi"("matrix type"=T3."General", "Input Matrix"=w489) -> ("determinant"=w497:dbl)  [unwired: 1 out]
                        n296 = Negate(x=w485) -> (-x=w488:dbl[])
                        n297 = Index Array(array=w485, index=0 ("disabled index (col)")) -> (element=w483:dbl)
                        n298 = Not Equal To 0?(x=w497) -> (x != 0?=w496:bool)
                        n299 = case shown="True" w496 {
                          tunnel: w489 -> [_ w528]
                          tunnel: w488 -> [_ w526]
                          tunnel: [9999999.9999 w508] -> w487
                          tunnel: [1.0 w514] -> w486
                          frame False {
                          }
                          frame True {
                            w521 = 0.25 ("x")
                            n300 = call-poly <vilib>:"Inverse Matrix.vi"("Input Matrix"=w528) -> ("Inverse Matrix"=w527:T7)  [unwired: 1 in, 1 out]
                            n301 = call-poly <vilib>:"A x B.vi"("Vector"=w526, "A"=w527) -> ("A x Vector"=w507:dbl[])  [unwired: 1 out]
                            n302 = Index Array(array=w507, index #1=0 ("index"), index #4=1 ("index")) -> (element #1=w515:dbl, element #2=w523:dbl, element #3=w517:dbl, element #4=w512:dbl)  [unwired: 2 in]
                            n303 = Square(x=w515) -> (x^2=w524:dbl)
                            n304 = Square(x=w523) -> (x^2=w522:dbl)
                            n305 = Sign(1:w515) -> (0:w514:dbl)
                            n306 = Multiply(x=w524, y=w521) -> (x*y=w520:dbl)
                            n307 = Multiply(x=w521, y=w522) -> (x*y=w519:dbl)
                            n308 = Add(x=w520, y=w519) -> (x+y=w518:dbl)
                            n309 = Multiply(x=w512, y=0.0) -> (x*y=w509:dbl)
                            n310 = Subtract(x=w518, y=w517) -> (x-y=w516:dbl)
                            n311 = Square Root(x=w516) -> (sqrt(x)=w510:dbl)
                            n312 = Add(x=w510, y=w509) -> (x+y=w508:dbl)
                          }
                        }
                      }
                      n313 = global read "G_VEH.vi" "C_Wheel base"() -> (w467:dbl)
                      n314 = Multiply(x=w475, y=w474) -> (x*y=w459:dbl[])
                      "x*y 2" <- w459
                      n315 = Square Root(x=w470) -> (sqrt(x)=w469:dbl[])
                      "sqrt(x)" <- w469
                      n316 = Threshold 1D Array(2:"y", 3:w469) -> (0:w471:dbl)  [unwired: 1 in]
                      n317 = Divide(x=w467, y=w459) -> (x/y=w466:dbl[])
                      n318 = Greater Or Equal To 0?(x="y") -> (x >= 0?=w472:bool)
                      n319 = Inverse Tangent(1:w466) -> (0:w465:dbl[])
                      n320 = case shown="True" w472 {
                        tunnel: w459 -> [_ w482]
                        tunnel: [w479 w481] -> w473
                        tunnel: w471 -> [_ w480]
                        frame False {
                          n321 = global read "G_VEH.vi" "Rtmp"() -> (w479:dbl)
                        }
                        frame True {
                          n322 = Interpolate 1D Array(1:w480, 2:w482) -> (0:w481:dbl)
                        }
                      }
                      n323 = Multiply(x=w465, y=180.0) -> (x*y=w463:dbl[])
                      n324 = global read "G_VEH.vi" "ratio_steer"() -> (w460:dbl)
                      n325 = Divide(x=w463, y=3.141592653589793) -> (x/y=w461:dbl[])
                      n326 = Multiply(x=w461, y=w460) -> (x*y=→"x*y":dbl[])
                    }
                  }
                  "map_track 2" <- w444
                }
                frame Enabled {
                  n327 = Array Size(array=w540) -> (size(s)=w547:i32[])
                  n328 = Index Array(array=w547, index=0) -> (element=w545:i32)
                  n329 = Subtract(x=w545, y=1) -> (x-y=w541:i32)
                  n330 = Greater Or Equal?(x=w541, y=1) -> (x >= y?=w542:bool)
                  n331 = case shown="True" w542 {
                    tunnel: w541 -> [_ w555]
                    tunnel: w540 -> [_ w554]
                    tunnel: [w551 w553] -> w530
                    tunnel: [w549 w552] -> w539
                    frame False {
                      n332 = Build Array(99999999.99) -> (w551:dbl[])
                      n333 = Build Array(6.0) -> (w549:dbl[])
                    }
                    frame True {
                      n334 = for {
                        N: w555 -> [_]
                        tunnel: w554 -> [w572]
                        tunnel: [w558] -> w553 mode=indexing
                        tunnel: [w556] -> w552 mode=indexing
                        i -> [w571]
                        n335 = Increment(x=w571) -> (x+1=w570:i32)
                        n336 = Index Array(array=w572, index (row) #1=w570, index (row) #2=w571) -> (element #1=w565:dbl[], element #2=w563:dbl[])  [unwired: 2 in]
                        n337 = Square(x=w565) -> (x^2=w568:dbl[])
                        n338 = Square(x=w563) -> (x^2=w567:dbl[])
                        n339 = Index Array(array=w565, index=0) -> (element=w560:dbl)
                        n340 = Index Array(array=w563, index=0) -> (element=w559:dbl)
                        n341 = Add Array Elements(numeric array=w568) -> (sum=w566:dbl)
                        n342 = Subtract(x=w560, y=w559) -> (x-y=w562:dbl)
                        n343 = Add Array Elements(numeric array=w567) -> (sum=w557:dbl)
                        n344 = Not Equal To 0?(x=w562) -> (x != 0?=w569:bool)
                        n345 = Square Root(x=w557) -> (sqrt(x)=w556:dbl)
                        n346 = case shown="True" w569 {
                          tunnel: w562 -> [_ w583]
                          tunnel: w557 -> [_ w590]
                          tunnel: w566 -> [_ w587]
                          tunnel: w560 -> [_ w589]
                          tunnel: w559 -> [_ w586]
                          tunnel: [99999999.99 w574] -> w558
                          frame False {
                          }
                          frame True {
                            n347 = Subtract(x=w587, y=w590) -> (x-y=w591:dbl)
                            n348 = Multiply(x=w590, y=w589) -> (x*y=w588:dbl)
                            n349 = Multiply(x=w587, y=w586) -> (x*y=w585:dbl)
                            n350 = Subtract(x=w588, y=w585) -> (x-y=w584:dbl)
                            n351 = Divide(x=w591, y=w583) -> (x/y=w577:dbl)
                            n352 = Divide(x=w584, y=w583) -> (x/y=w579:dbl)
                            n353 = Square(x=w577) -> (x^2=w582:dbl)
                            n354 = Multiply(x=w582, y=0.25) -> (x*y=w580:dbl)
                            n355 = Subtract(x=w580, y=w579) -> (x-y=w578:dbl)
                            n356 = Sign(1:w577) -> (0:w575:dbl)
                            n357 = Square Root(x=w578) -> (sqrt(x)=w576:dbl)
                            n358 = Multiply(x=w575, y=w576) -> (x*y=w574:dbl)
                          }
                        }
                      }
                    }
                  }
                  "Array" <- w530
                  "Array 2" <- w539
                  n359 = global read "G_VEH.vi" "C_Wheel base"() -> (w538:dbl)
                  n360 = Divide(x=w538, y=w530) -> (x/y=w537:dbl[])
                  n361 = Inverse Tangent(1:w537) -> (0:w536:dbl[])
                  n362 = Multiply(x=w536, y=180.0) -> (x*y=w534:dbl[])
                  n363 = global read "G_VEH.vi" "ratio_steer"() -> (w531:dbl)
                  n364 = Divide(x=w534, y=3.141592653589793) -> (x/y=w532:dbl[])
                  n365 = Multiply(x=w532, y=w531) -> (x*y=→"Waveform Graph":dbl[])
                }
              }
            }
          }
          "R" <- w305
        }
      }
    }
  }
